vi "IniDataRd RS485.vi"(8 "error in":errorcluster, 10 "RS485 section":string="RS485 MachiningRoom", 11 "INI file path":path=path "D:/DSA 開發課/1.開發專案/WDB13/Labview/WDB10 Labview/ref/IniData.ini") -> (0 "error out":errorcluster, 2 "RS485 para":T1={"Com"="", "Baud Rate"=8193, "Parity"=0} {"Parity" items=["None", "Odd", "Even", "Mark", "Space"]})   [LabVIEW 2019]
uses:
  <vilib>/Utility/config.llb/Read Key (String).vi
  <vilib>/Utility/config.llb/Read Key (U32).vi
  <vilib>/Utility/config.llb/NI_LVConfig.lvlib
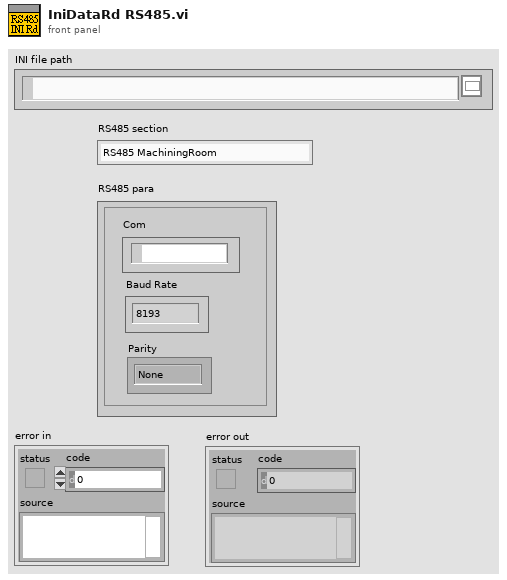
[diagram p1: front panel]
types:
  T1 = cluster{"Com":refnum<visa-resource-name>, "Baud Rate":u32, "Parity":u16}
  T2 = typedef "NI_LVConfig.lvlib/Config Data RefNum.ctl" = refnum<k1>
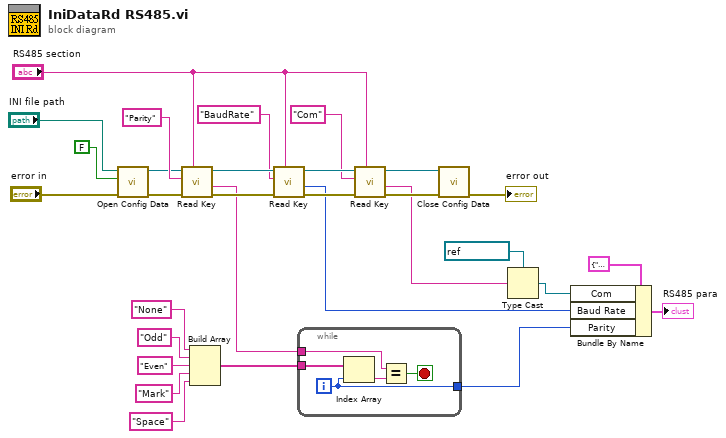
[diagram p0: block diagram]
diagram:
  n1 = call <vilib>:"Open Config Data.vi"("error in (no error)"="error in", "create file if necessary (T)"=FALSE ("create file if necessary? (T)"), "configuration file path"="INI file path") -> ("error out"=w28:errorcluster, "refnum"=w26:T2)  [unwired: 6 in, 1 out]
  n2 = call-poly <vilib>:"Read Key.vi"("section"="RS485 section", "error in (no error)"=w28, "key"="Parity", "refnum"=w26) -> ("error out"=w21:errorcluster, "value"=w8:string, "refnum out"=w25:T2)  [unwired: 2 in, 3 out]
  n3 = Build Array("None", "Odd", "Even", "Mark", "Space") -> (w2:string[])
  n4 = call-poly <vilib>:"Read Key.vi"("section"="RS485 section", "error in (no error)"=w21, "key"="BaudRate", "refnum"=w25) -> ("error out"=w20:errorcluster, "value"=w10:u32, "refnum out"=w23:T2)  [unwired: 1 in, 4 out]
  n5 = while {
    tunnel: w8 -> [w34]
    tunnel: w2 -> [w35]
    tunnel: [w31] -> w1
    i -> [w31]
    stop <- w32 stop-if-true
    n6 = Index Array(array=w35, index=w31) -> (element=w33:string)
    n7 = Equal?(x=w34, y=w33) -> (x = y?=w32:bool)
  }
  n8 = call-poly <vilib>:"Read Key.vi"("section"="RS485 section", "error in (no error)"=w20, "key"="Com", "refnum"=w23) -> ("error out"=w19:errorcluster, "value"=w13:string, "refnum out"=w22:T2)  [unwired: 2 in, 3 out]
  n9 = call <vilib>:"Close Config Data.vi"("error in (no error)"=w19, "refnum"=w22) -> ("error out"=→"error out":errorcluster)  [unwired: 1 in, 8 out]
  n10 = Type Cast(type=refnum<visa-resource-name> "COM7" ("VISA resource name"), x=w13) -> (*(type *) &x=w9:refnum<visa-resource-name>)
  n11 = Bundle By Name(cluster=T1 {"Com"="", "Baud Rate"=8193, "Parity"=3} ("RS485 para"), "Com"=w9, "Baud Rate"=w10, "Parity"=w1) -> (→"RS485 para":T1)
